vi "读文件main.vi"(11 "VISA资源名称":refnum<visa-resource-name>="COM3") -> (0 "消息":string, 2 "数据":string[][](array[string]), 3 "VISA资源名称 2":refnum<visa-resource-name>)   [LabVIEW 2015]
uses:
  Globle.vi
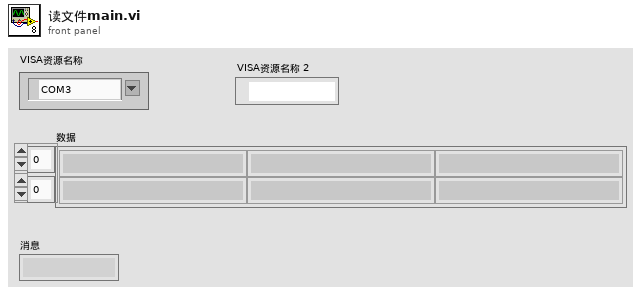
[diagram p1: front panel]
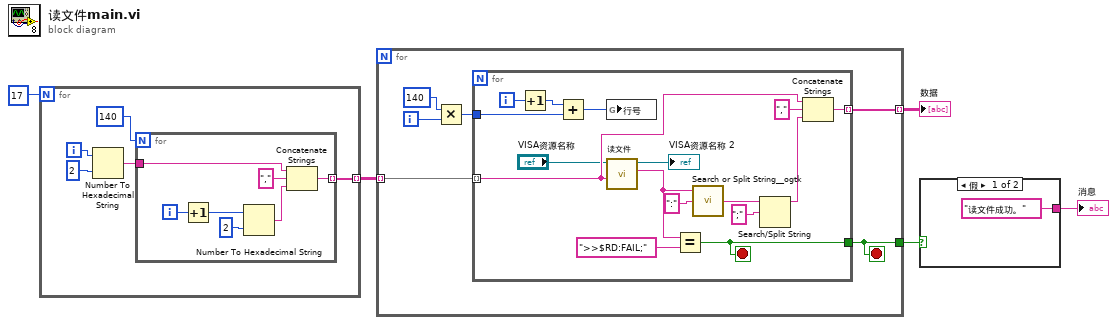
[diagram p0: block diagram]
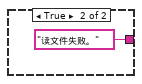
[diagram p2: hidden frame]
diagram:
  n1 = for {
    N: 17 -> [_]
    tunnel: [w6] -> w4 mode=indexing
    i -> [w10]
    n2 = Number To Hexadecimal String(1:i16 2 ("宽度(-)"), 2:w10) -> (0:w7:string)
    n3 = for {
      N: 140 -> [_]
      tunnel: w7 -> [w12]
      tunnel: [w13] -> w6 mode=indexing
      i -> [w17]
      n4 = Increment(x=w17) -> (x+1=w15:i32)
      n5 = Number To Hexadecimal String(1:i16 2 ("宽度(-)"), 2:w15) -> (0:w11:string)
      n6 = Concatenate Strings(w12, "," ("字符串"), w11) -> (w13:string)
    }
  }
  n7 = for {
    tunnel: w4 -> [w23] mode=indexing
    tunnel: [w22] -> w3
    tunnel: [w21] -> w2 mode=indexing
    i -> [w20]
    stop <- w22 stop-if-true
    n8 = Multiply(x=140, y=w20) -> (x*y=w18:i32)
    n9 = for {
      tunnel: w23 -> [w33] mode=indexing
      tunnel: [w38] -> w22
      tunnel: [w31] -> w21 mode=indexing
      tunnel: w18 -> [w25]
      i -> [w27]
      stop <- w38 stop-if-true
      n10 = Increment(x=w27) -> (x+1=w26:i32)
      n11 = Add(x=w26, y=w25) -> (x+y=w24:i32)
      n12 = global write "Globle.vi" "行号"(w24) -> ()
      n13 = call "读文件.vi"("参数"=w33, "VISA资源名称"="VISA资源名称") -> ("响应"=w36:string, "VISA资源名称 2"=→"VISA资源名称 2":refnum<visa-resource-name>)  [unwired: 8 in]
      n14 = Equal?(x=w36, y=">>$RD:FAIL;") -> (x = y?=w38:bool)
      n15 = call <userlib>:"Search or Split String__ogtk.vi"("search string/char (-)"=":", "string"=w36) -> ("substring after match"=w34:string)  [unwired: 1 in, 2 out]
      n16 = Search/Split String(string=w34, search string/char (-)=";" ("搜索字符串/字符(-)")) -> (substring before match=w28:string)  [unwired: 1 in, 2 out]
      n17 = Concatenate Strings(w33, "," ("字符串"), w28) -> (w31:string)
    }
  }
  "数据" <- w2
  n18 = case shown="假" w3 {
    tunnel: ["读文件成功。" "读文件失败。"] -> w1
    frame False {
    }
    frame True {
    }
  }
  "消息" <- w1
